vi "读取输入状态.vi"(8 "error in (no error)":errorcluster, 10 "Slave ID":u8=1, 11 "MB session in":refnum<class "MB_Master.lvclass">) -> (0 "error out":errorcluster, 2 "Coils":bool[](array[boolean]), 3 "MB session out":refnum<class "MB_Master.lvclass">)   [LabVIEW 2016, in "斯坦道功率测流.lvlib"]
uses:
  <vilib>/Plasmionique/MB Master/MB_Master/MB_Master.lvclass
  <vilib>/Plasmionique/MB Master/MB Master.lvlib
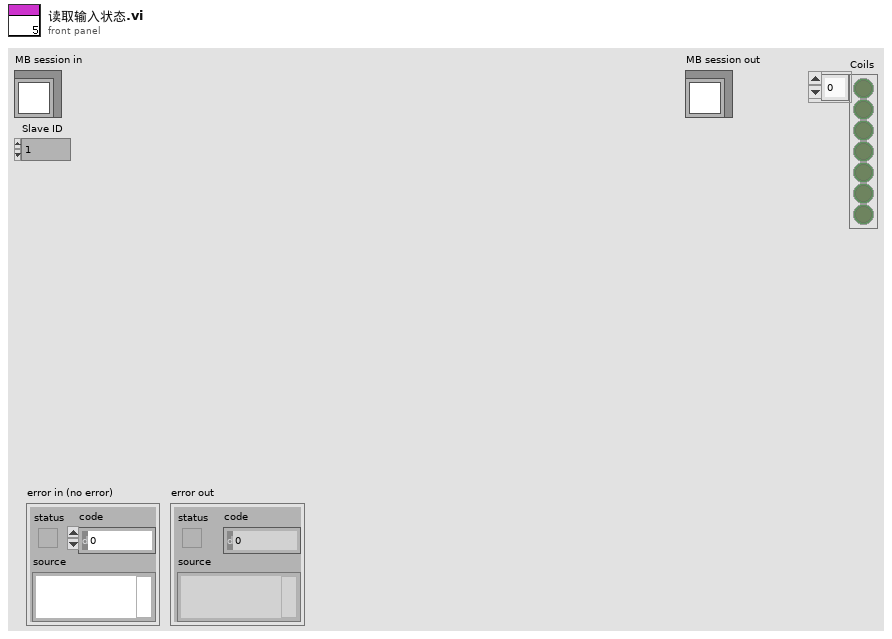
[diagram p1: front panel]
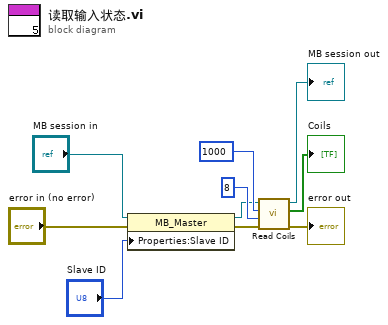
[diagram p0: block diagram]
diagram:
  n1 = property class="MB_Master"(reference="MB session in", error in="error in (no error)", "Properties:Slave ID"="Slave ID") -> (reference out=w5:refnum<class "MB_Master.lvclass">, error out=w3:errorcluster)
  n2 = call <vilib>:"Read Coils.vi"("error in (no error)"=w3, "quantity"=u16 8, "starting address"=u16 1000, "MB session in"=w5) -> ("error out"=→"error out":errorcluster, "Coils"=→"Coils":bool[], "MB session out"=→"MB session out":refnum<class "MB_Master.lvclass">)  [unwired: 5 in]
